vi "VI Server_SingleInstanceSelector.vi"(2 "Single Instance (T)":bool=TRUE) -> (6 "Single Instance.OUT":bool)   [LabVIEW 2020, in "VI Server Toolkit LV2013.lvlib"]
doc: "Returns if there was first call of the calling VI and how it should be used.\nMostly used in Set Controls and Get Controls VI of the VI Server Toolkit in order to avoid repeating of the search and index controls references arrays and convert reference from generic into data type specific format."
uses:
  VI Server Toolkit LV2013.lvlib
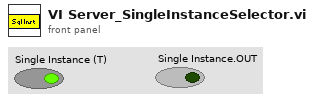
[diagram p1: front panel]
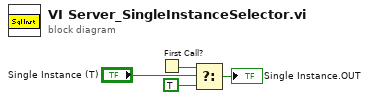
[diagram p0: block diagram]
diagram:
  n1 = First Call?() -> (First Call?: T/F=w1:bool)
  n2 = Select(t=w1, s="Single Instance (T)", f=TRUE) -> (s? t:f=→"Single Instance.OUT":bool)
